vi "FileString To Base64.vi"(8 "error in (no error)":errorcluster, 9 "String":string, 10 "文件（使用对话框）":path=path "C:/Users/wangzhen/Desktop/BaiduFaceAPI_For_Labview-master（人脸识别）/BaiduFaceAPI_For_Labview-master/test Images/5.jpg", 11 "Action":enum16{"EncodeString", "EcodeFile"}(ring)) -> (0 "error out":errorcluster, 1 "长度":i32, 2 "string out (base64-encoded)":string, 3 "encodeURIComponent":string)   [LabVIEW 2017, in "Encode Base64.lvlib"]
uses:
  Encode Base64.lvlib
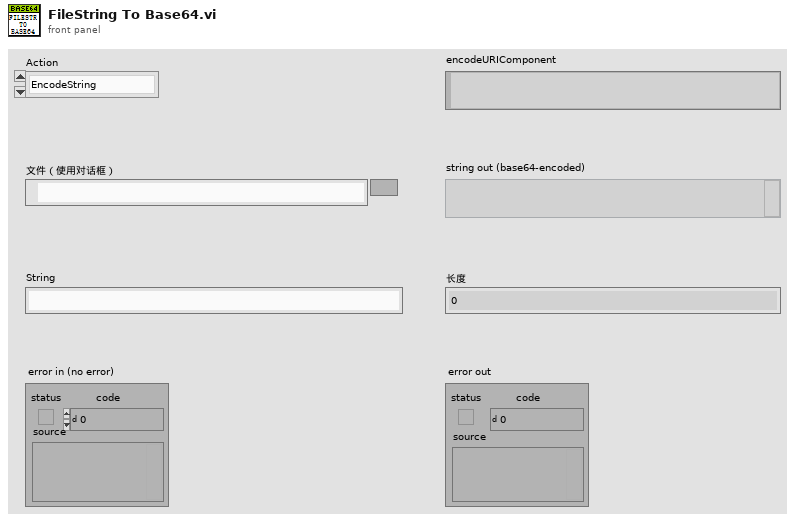
[diagram p1: front panel]
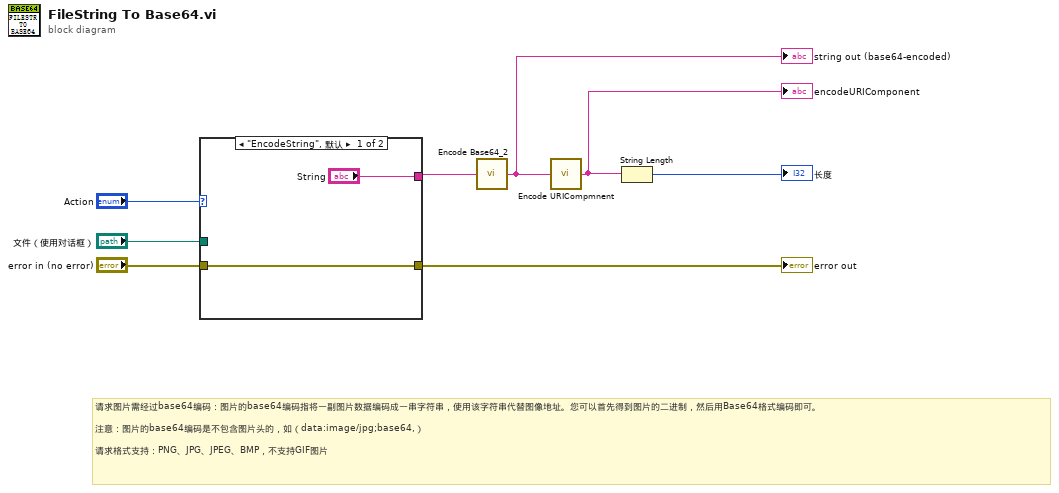
[diagram p0: block diagram]
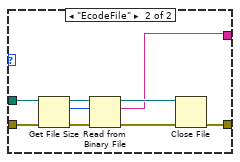
[diagram p2: hidden frame]
diagram:
  # "请求图片需经过base64编码：图片的base64编码指将一副图片数据编码成一串字符串，使用该字符串代替图像地址。您可以首先得到图片的二进制，然后用Base64格式编码即可。\n\n注意：图片的base64编码是不包含图片头的，如（data:image/jpg;base64,）\n\n请求格式支持：PNG、JPG、JPEG、BMP，不支持GIF图片"
  n1 = case shown="\"EncodeString\", 默认" "Action" {
    tunnel: "文件（使用对话框）" -> [_ w19]
    tunnel: ["String" w13] -> w7
    tunnel: [w10 w12] -> w5
    tunnel: "error in (no error)" -> [w10 w11]
    frame "EncodeString", Default {
    }
    frame "EcodeFile" {
      n2 = Get File Size(file=w19, error in=w11) -> (refnum out=w18:refnum<file>, size (in bytes)=w17:i64, 0:w16:errorcluster)
      n3 = Read from Binary File(8:w16, 10:w17, 11:w18) -> (0:w14:errorcluster, 2:w13:string, 3:w15:refnum<file>)  [unwired: 3 in, 1 out]
      n4 = Close File(refnum=w15, error in=w14) -> (error out=w12:errorcluster)  [unwired: 1 out]
    }
  }
  "error out" <- w5
  n5 = call "Encode Base64_2.vi"("string in (not encoded)"=w7) -> ("string out (base64-encoded)"=w6:string)
  "string out (base64-encoded)" <- w6
  n6 = call "Encode URICompmnent.vi"("URI"=w6) -> ("encodeURIComponent"=w3:string)
  "encodeURIComponent" <- w3
  n7 = String Length(string=w3) -> (length=→"长度":i32)
